vi "GRPCClientExample.vi"() -> ()   [LabVIEW 2019, in "MicronGRPCClient.lvclass"]
uses:
  MicronGRPCClient.lvclass
  Base/Client/MicronClient.lvclass
panel:
  in  "Connection Type":enum32{"Start New", "Connect Existing"}(tab)=enum."Connect Existing"
  in  "Path":path=path "../Builds/GRPC/Server/GRPCServerExample.exe"
  in  "Connection String":string="localhost:50051"
  out "error out":errorcluster
  out "Response":string
  in  "Command":string="Hello World!"
  in  "Payload":string="Popping in to say hi!"
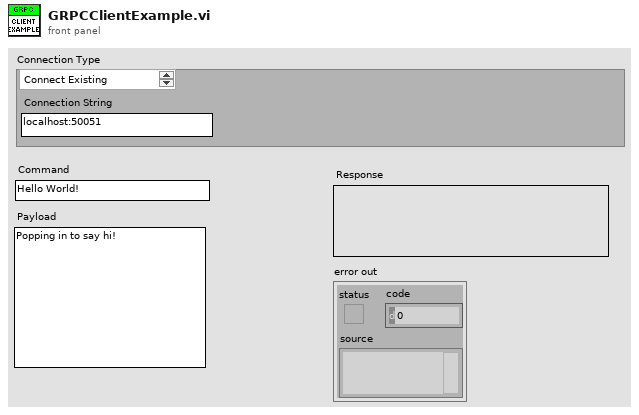
[diagram p1: front panel]
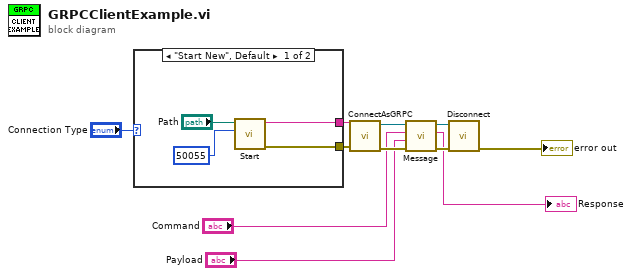
[diagram p0: block diagram]
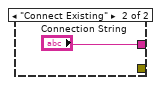
[diagram p2: hidden frame]
diagram:
  n1 = case shown="\"Start New\", Default" "Connection Type" {
    tunnel: [w12 _] -> w3
    tunnel: [w15 "Connection String"] -> w2
    frame "Start New", Default {
      n2 = call "Start.vi"("Port"=50055, "Micron Path"="Path") -> ("error out"=w12:errorcluster, "Connection String"=w15:string)  [unwired: 8 in]
    }
    frame "Connect Existing" {
    }
  }
  n3 = call "ConnectAsGRPC.vi"("error in"=w3, "Connection String"=w2) -> ("error out"=w11:errorcluster, "MicronClient out"=w10:refnum<class "MicronClient.lvclass">)  [unwired: 8 in]
  n4 = call-dynamic "Message.vi"("error in (no error)"=w11, "Payload"="Payload", "Command"="Command", "MicronClient in"=w10) -> ("error out"=w8:errorcluster, "Response"=→"Response":string, "MicronClient out"=w9:refnum<class "MicronClient.lvclass">)  [unwired: 5 in]
  n5 = call-dynamic "Disconnect.vi"("error in (no error)"=w8, "MicronClient in"=w9) -> ("error out"=→"error out":errorcluster)  [unwired: 8 in, 1 out]
